vi "toTReKGPS-Epoch.vi"(11 "Epoch in":refnum<class "Epoch.UTC.lvclass">) -> (2 "TReK GPS Epoch Time":fxp<+,32,32>, 3 "Epoch":refnum<class "Epoch.UTC.lvclass">)   [LabVIEW 2013]
uses:
  Epoch.UTC.lvclass
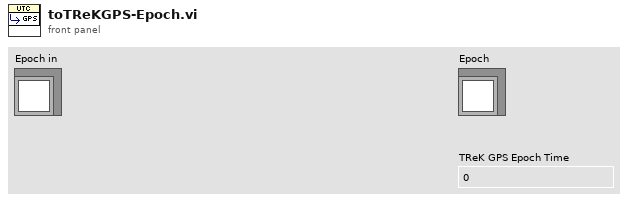
[diagram p1: front panel]
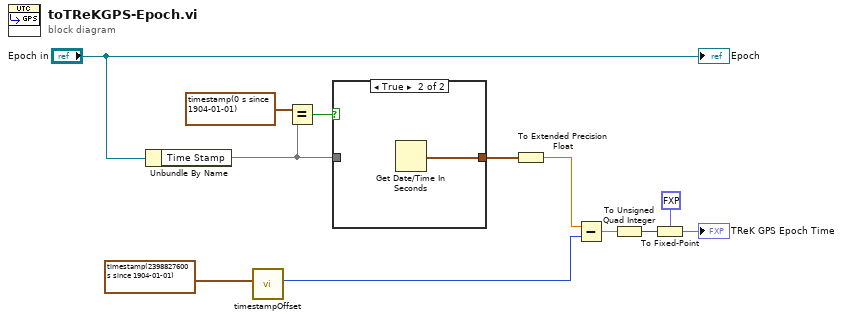
[diagram p0: block diagram]
diagram:
  n1 = Unbundle By Name("Epoch in") -> ("Time Stamp"=w4)
  n2 = call "timestampOffset.vi"("Reference Time"=timestamp(2398827600 s since 1904-01-01) ("Timestamp")) -> ("Timestamp Offset"=w8:i64)  [unwired: 10 in]
  n3 = Equal?(x=timestamp(0 s since 1904-01-01), y=w4) -> (x = y?=w6:bool)
  n4 = case shown="True" w6 {
    tunnel: [w13 w14] -> w5
    tunnel: w4 -> [w13 _]
    frame False {
    }
    frame True {
      n5 = Get Date/Time In Seconds() -> (seconds since 1Jan1904=w14:timestamp)
    }
  }
  n6 = To Extended Precision Float(1:w5) -> (0:w10:ext)
  n7 = Subtract(x=w10, y=w8) -> (x-y=w11:ext)
  n8 = To Unsigned Quad Integer(1:w11) -> (0:w3:u64)
  n9 = To Fixed-Point(fixed-point type=fxp<+,32,32> 0.0 ("TReK GPS Epoch Time"), number=w3) -> (fixed-point=→"TReK GPS Epoch Time":fxp<+,32,32>)
  "Epoch" <- "Epoch in"
